vi "_[error50003]Default Config File Name Error.vi"(8 "error in (no error)":errorcluster) -> (0 "error out":errorcluster)   [LabVIEW 2017, in "TagDB.lvlib"]
uses:
  TagDB.lvlib
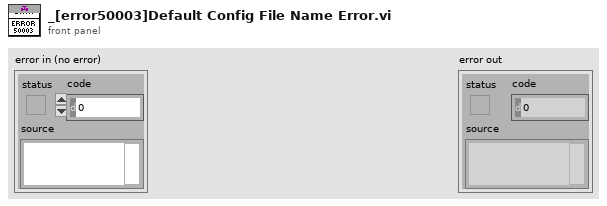
[diagram p1: front panel]
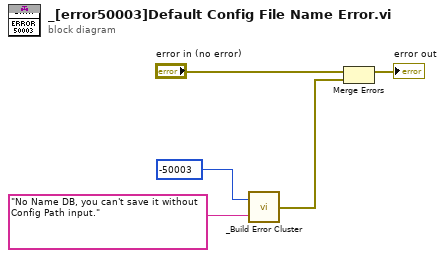
[diagram p0: block diagram]
diagram:
  n1 = call "_Build Error Cluster.vi"("String to Prepend to source (\"\")"="No Name DB, you can't save it without Config Path input." ("source"), "code"=-50003) -> ("error out"=w2:errorcluster)
  n2 = Merge Errors("error in (no error)", w2) -> (→"error out":errorcluster)
